vi "Introspection Core.vi"(8 "error in (no error)":errorcluster, 11 "CS++IEFWerner in":refnum<class "CS++IEFWerner.lvclass">) -> (0 "error out":errorcluster, 2 "CS++Messages":refnum<class "Message.lvclass">[](array[class]), 3 "CS++IEFWerner out":refnum<class "CS++IEFWerner.lvclass">)   [LabVIEW 2015, in "CS++IEFWerner.lvlib" / "CS++IEFWerner.lvclass"]
doc: "This vi delivers a list with all messages this actor reacts to. \n\nNote that all inherited classes have to overwrite it."
uses:
  CS++IEFWerner.lvclass
  <vilib>/ActorFramework/Message/Message.lvclass
  CS++IEFWerner Messages/Update_Readback Msg/Update_Readback Msg.lvclass
  CSPP_DeviceBase/CS++Motor/CS++Motor.lvclass
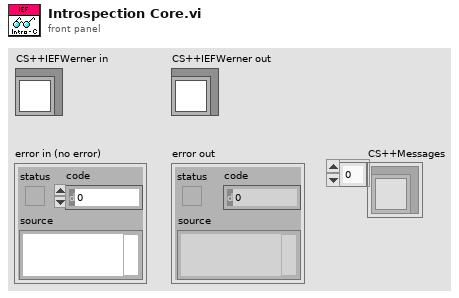
[diagram p1: front panel]
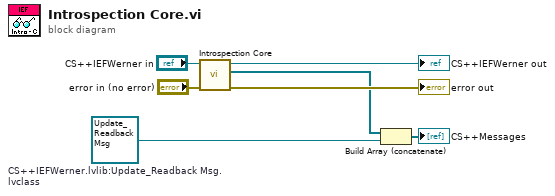
[diagram p0: block diagram]
diagram:
  w1 = refnum<class "Update_Readback Msg.lvclass"> refnum  # CS++IEFWerner.lvlib:Update_Readback Msg.lvclass
  n1 = call-parent "Introspection Core.vi"("error in (no error)"="error in (no error)", "CS++Motor in"="CS++IEFWerner in") -> ("error out"=→"error out":errorcluster, "CS++Messages"=w3:refnum<class "Message.lvclass">[], "CS++Motor out"=→"CS++IEFWerner out":refnum<class "CS++IEFWerner.lvclass">)  [unwired: 7 in]
  n2 = Build Array (concatenate)(w3, w1) -> (→"CS++Messages":refnum<class "Message.lvclass">[])
